vi "Add Pressure Channels.vi"(11 "Array in":T1=[0.0, 0.0, 0.0, 0.0, 0.0, 0.0, 0.0, 0.0, 0.0, 0.0, 0.0, 0.0, 0.0, 0.0, 0.0, 0.0, 0.0, 0.0, 0.0, 0.0, 0.0, 0.0, 0.0, 0.0, 0.0, 0.0, 0.0, 0.0, 0.0, 0.0, 0.0, 0.0, 0.0, 0.0, 0.0, 0.0, 0.0, 0.0, 0.0, 0.0, 0.0, 0.0, 0.0, 0.0, 0.0, 0.0, 0.0, 0.0, 0.0, 0.0]) -> (3 "Array Out":T2)   [LabVIEW 2022 SP3]
doc: "Author: Scott Hannahs <sth@magnet.fsu.edu>\nCopyright 2018 Florida State University, All rights reserved."
uses:
  SCH Data Controls/SCH Int Data with Pressure.ctl
  SCH Data Controls/SCH All FXP Data.ctl
  <vilib>/rvi/eio/common/nirviEmuTemplateMethod_errors.vi
  <vilib>/eio/EIONode/EIONode.xnode
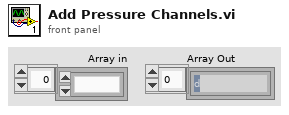
[diagram p1: front panel]
types:
  T1 = typedef "SCH All FXP Data.ctl" = fxp<+/-,19,5>[]
  T2 = typedef "SCH Int Data with Pressure.ctl" = fxp<+/-,19,5>[]
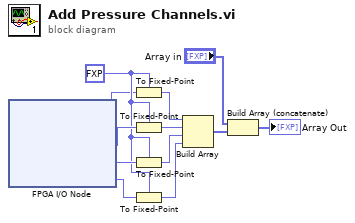
[diagram p0: block diagram]
diagram:
  w2 = fxp<+/-,19,5> 0.0 ("fixed-point type")
  n1 = xnode "FPGA I/O Node"() -> ("PI751 Inlet"=w1:fxp<+/-,24,5>, "PI752 Inlet"=w10:fxp<+/-,24,5>, "PI753 Inlet"=w9:fxp<+/-,24,5>, "PI755 Outlet"=w8:fxp<+/-,24,5>)  [unwired: 4 in, 4 out]
  n2 = To Fixed-Point(fixed-point type=w2, number=w1) -> (fixed-point=w6:fxp<+/-,19,5>)
  n3 = To Fixed-Point(fixed-point type=w2, number=w10) -> (fixed-point=w5:fxp<+/-,19,5>)
  n4 = To Fixed-Point(fixed-point type=w2, number=w9) -> (fixed-point=w4:fxp<+/-,19,5>)
  n5 = To Fixed-Point(fixed-point type=w2, number=w8) -> (fixed-point=w3:fxp<+/-,19,5>)
  n6 = Build Array(w6, w5, w4, w3) -> (w7:fxp<+/-,19,5>[])
  n7 = Build Array (concatenate)("Array in", w7) -> (→"Array Out":fxp<+/-,19,5>[])
